vi "test.vi"() -> ()   [LabVIEW 2015]
uses:
  <vilib>/measure/matone.llb/SINAD Analyzer 1 Chan.vi
  <vilib>/measure/NI_MAPro.lvlib
panel:
  in  "分析通道":u16(ring) items=["0", "1", "2", "3"]
  out "导出的信号频谱(dBV)":T1(graph)
  out "THD Plus Noise":dbl caption="总谐波失真叠加噪声" format="%.2p"
  out "SINAD (dB)":dbl format="%.2p"
  out "detected fundamental\nfrequency":dbl caption="检测出的基频" format="%.2p"
  out "波形图3":i16[](graph)
  out "波形图2":i16[](graph)
  out "波形图1":i16[](graph)
  out "波形图0":i16[](graph)
  in  "路径":path
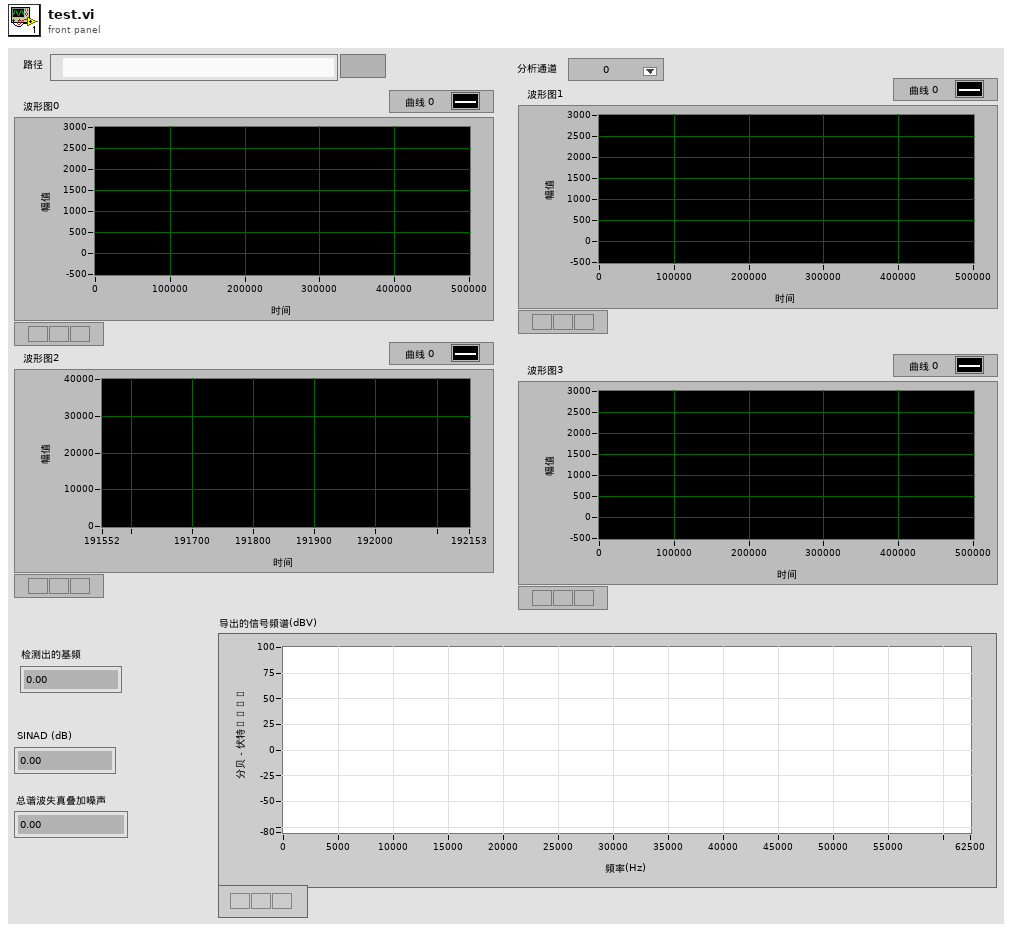
[diagram p1: front panel]
types:
  T1 = cluster{"f0":dbl, "df":dbl, "dB Spectrum (Hann)":dbl[]}
  T2 = enum16{"none", "input signal", "fundamental signal", "residual signal"}
  T3 = enum16{"big-endian, network order", "native, host order", "little-endian"}
  T4 = enum16{"open", "replace", "create", "open or create", "replace or create", "replace or create with confirmation"}
  T5 = cluster{"exported time signal":waveform(dbl), "exported spectrum (dB)":cluster{"f0":dbl, "df":dbl, "dB Spectrum (Hann)":dbl[]}}
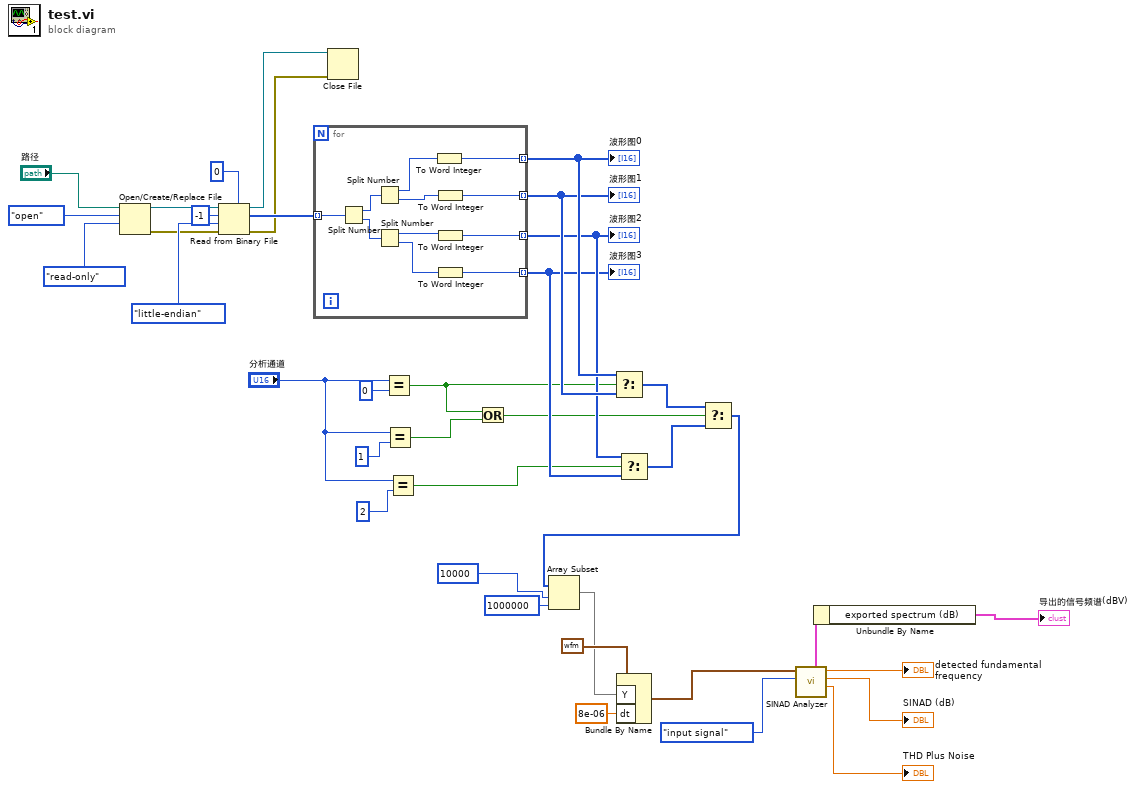
[diagram p0: block diagram]
diagram:
  n1 = Open/Create/Replace File(file path (use dialog)="路径", operation (0:open)=T4."open" ("操作(0:open)"), access (0:read/write)=enum16{"read/write", "read-only", "write-only"}."read-only" ("权限(0:read/write)")) -> (refnum out=w36:refnum<file>, error out=w33:errorcluster)  [unwired: 3 in, 1 out]
  n2 = Read from Binary File(5:u64 0, 8:w33, 9:T3."little-endian" ("字节顺序(0:big-endian, network order)"), 10:-1 ("总数(1)"), 11:w36) -> (0:w28:errorcluster, 2:w31:u64[], 3:w29:refnum<file>)  [unwired: 1 in, 1 out]
  n3 = for {
    tunnel: w31 -> [w49] mode=indexing
    tunnel: [w42] -> w16 mode=indexing
    tunnel: [w41] -> w15 mode=indexing
    tunnel: [w40] -> w14 mode=indexing
    tunnel: [w39] -> w13 mode=indexing
    n4 = Split Number(x=w49) -> (hi(x)=w48:u32, lo(x)=w47:u32)
    n5 = Split Number(x=w48) -> (hi(x)=w46:u16, lo(x)=w45:u16)
    n6 = Split Number(x=w47) -> (hi(x)=w43:u16, lo(x)=w44:u16)
    n7 = To Word Integer(number=w46) -> (16bit integer=w42:i16)
    n8 = To Word Integer(number=w45) -> (16bit integer=w41:i16)
    n9 = To Word Integer(number=w43) -> (16bit integer=w40:i16)
    n10 = To Word Integer(number=w44) -> (16bit integer=w39:i16)
  }
  "波形图0" <- w16
  "波形图1" <- w15
  "波形图2" <- w14
  "波形图3" <- w13
  n11 = Close File(refnum=w29, error in=w28) -> ()  [unwired: 2 out]
  n12 = Equal?(x="分析通道", y=u16 0) -> (x = y?=w7:bool)
  n13 = Equal?(x="分析通道", y=u16 1) -> (x = y?=w6:bool)
  n14 = Equal?(x="分析通道", y=u16 2) -> (x = y?=w2:bool)
  n15 = Or(x=w7, y=w6) -> (x .or. y?=w5:bool)
  n16 = Select(t=w16, s=w7, f=w15) -> (s? t:f=w12:i16[])
  n17 = Select(t=w14, s=w2, f=w13) -> (s? t:f=w11:i16[])
  n18 = Select(t=w12, s=w5, f=w11) -> (s? t:f=w10:i16[])
  n19 = Array Subset(array=w10, index=10000 ("长度"), length=1000000 ("长度")) -> (w17:i16[])
  n20 = Bundle By Name(cluster=waveform(dbl) {"t0"=timestamp(0 s since 1904-01-01), "dt"=1.0, "Y"=[]} ("signal in"), "Y"=w17, "dt"=8e-06) -> (w22:waveform(dbl))
  n21 = call-poly <vilib>:"SINAD Analyzer.vi"("export  mode"=T2."input signal", "signal in"=w22) -> ("THD Plus Noise"=→"THD Plus Noise":dbl, "SINAD (dB)"=→"SINAD (dB)":dbl, "detected fundamental\nfrequency"=→"detected fundamental\nfrequency":dbl, "exported signals"=w21:T5)  [unwired: 4 in, 2 out]
  n22 = Unbundle By Name(w21) -> ("exported spectrum (dB)"=→"导出的信号频谱(dBV)":T1)
